vi "Create AI Mode.vi"(7 "mode settings":variant, 8 "error in":errorcluster, 9 "number of channels":i32, 10 "channel settings":T1[](array[typedef]), 11 "mode in":refnum<class "Analog Input Mode.lvclass">) -> (0 "error out":errorcluster, 1 "channels":refnum<class "AI Channel.lvclass">[](array[class]), 3 "mode out":refnum<class "Analog Input Mode.lvclass">)   [LabVIEW 2017, in "Scan Engine Scripting.lvlib" / "Analog Input Mode.lvclass"]
uses:
  Analog Input Vrms Mode/Analog Input Mode.lvclass
  Channel Classes/AI Channel/AI Channel.lvclass
  Controls/analog channel settings.ctl
  Scan Engine Scripting.lvlib
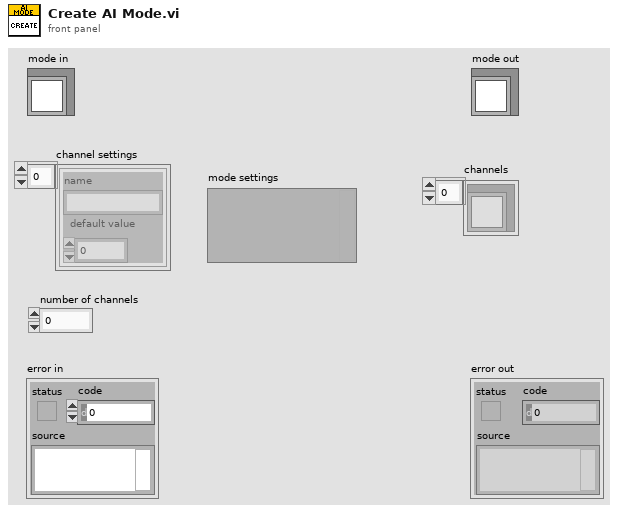
[diagram p1: front panel]
types:
  T1 = typedef "Scan Engine Scripting.lvlib/analog channel settings.ctl" = cluster{"name":string, "default value":dbl}
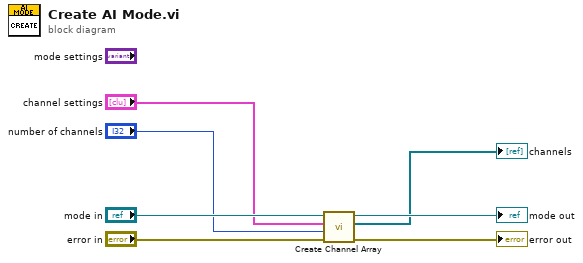
[diagram p0: block diagram]
diagram:
  n1 = call "Create Channel Array.vi"("error in"="error in", "expected channel count"="number of channels", "channel settings"="channel settings", "analog input mode in"="mode in") -> ("error out"=→"error out":errorcluster, "channels"=→"channels":refnum<class "AI Channel.lvclass">[], "analog input mode out"=→"mode out":refnum<class "Analog Input Mode.lvclass">)  [unwired: 5 in]
